vi "cBRS Readout.vi"() -> ()   [LabVIEW 2018]
uses:
  <vilib>/Utility/error.llb/DialogType.ctl
  <vilib>/DAQmx/read.llb/DAQmx Read (Analog 1D Wfm NChan NSamp).vi
  <vilib>/DAQmx/write.llb/DAQmx Write (Analog DBL 1Chan 1Samp).vi
  <vilib>/DAQmx/create/channels.llb/DAQmx Create Channel (AI-Voltage-Basic).vi
  <vilib>/DAQmx/configure/timing.llb/DAQmx Timing (Sample Clock).vi
  <vilib>/DAQmx/create/channels.llb/DAQmx Create Channel (AO-Voltage-Basic).vi
  <vilib>/DAQmx/miscellaneous.llb/DAQmx Fill In Error Info.vi
panel:
  in  "Capacitor Feedback":bool
  in  "Piezo Feedback":bool
  in  "Gain 1":dbl
  in  "Physical Channel 5":tag="Dev1/ao3" caption="Physical Channel"
  in  "Physical Channel 4":tag="Dev1/ao2" caption="Physical Channel"
  in  "I Reset 2":bool
  in  "I Reset 1":bool
  in  "To Disk Freq":dbl=500.0 caption="dt"
  in  "DC Offset 2":dbl
  in  "I term 2":dbl=5000.0
  in  "Gain 2":dbl=0.005
  in  "Setpoint 2":dbl=5.0
  in  "Physical Channel 3":tag="Dev1/ao1" caption="Physical Channel"
  in  "I term":dbl=5000.0
  in  "Output terminal configuration":i32(ring)=10083 items=["Default"=-1, "RSE"=10083, "Differential"=10106, "Pseudodifferential"=12529]
  in  "DC Offset":dbl
  in  "Gain":dbl=0.005
  in  "Setpoint":dbl=5.0
  in  "Physical Channel 2":tag="Dev1/ao0" caption="Physical Channel"
  in  "Input terminal configuration":i32(ring)=10106 items=["default"=-1, "RSE"=10083, "NRSE"=10078, "Differential"=10106, "Pseudodifferential"=12529]
  in  "Down Sample Freq":dbl=1000.0 caption="dt"
  out "Waveform Chart":dynamicdata(graph)=[{"t0"=timestamp(3662756182.4372287 s since 1904-01-01), "dt"=1.9999999999999998e-05, "Y"=array[500 elements], "attributes"=variant("NI_ChannelName"=variant(string "Dev1/ai0"), "NI_UnitDescription"=variant(string "Volts"))}, {"t0"=timestamp(3662756182.4372387 s since 1904-01-01), "dt"=1.9999999999999998e-05, "Y"=array[500 elements], "attributes"=variant("NI_ChannelName"=variant(string "Dev1/ai2"), "NI_UnitDescription"=variant(string "Volts"))}, {"t0"=timestamp(3662756182.4372287 s since 1904-01-01), "dt"=0.001, "Y"=[0.0, 0.0, 0.0, 0.0, 0.0, 0.0, 0.0, 0.0, 0.0, 0.0], "attributes"=variant("NI_ChannelName"=variant(string "Dev1/ai0 (Filtered)"), "NI_OriginalChannelName"=variant(string "Dev1/ai0"), "NI_UnitDescription"=variant(string "Volts"))}, {"t0"=timestamp(3662756182.4372287 s since 1904-01-01), "dt"=0.001, "Y"=[0.0, 0.0, 0.0, 0.0, 0.0, 0.0, 0.0, 0.0, 0.0, 0.0], "attributes"=variant("NI_ChannelName"=variant(string "Dev1/ai2 (Filtered)"), "NI_OriginalChannelName"=variant(string "Dev1/ai2"), "NI_UnitDescription"=variant(string "Volts"))}, {"t0"=timestamp(3662756182.4372287 s since 1904-01-01), "dt"=0.001, "Y"=[3.746254926547408, 3.7462550457566977, 3.7462551556527615, 3.746255255304277, 3.7462553502991796, 3.746255445294082, 3.7462555365636945, 3.7462556241080165, 3.7462557135149837, 3.7462558085098863], "attributes"=variant("NI_ChannelName"=variant(string "Dev1/ai0 (Filtered)"), "NI_OriginalChannelName"=variant(string "Dev1/ai0"), "NI_UnitDescription"=variant(string "Volts"))}]
  in  "Write":bool caption="Enable"
  in  "stop":bool
  in  "Samples to Read":i32=500
  in  "Sample Rate":dbl=50000.0 caption="Read Rate (Hz)" format="%0.2f"
  in  "Physical Channel":tag="Dev1/ai0, Dev1/ai2" caption="Input Physical Channel"
  # "Piezo Feedback 1"
  # "Piezo Feedback 2"
  # "Capacitor Feedback"
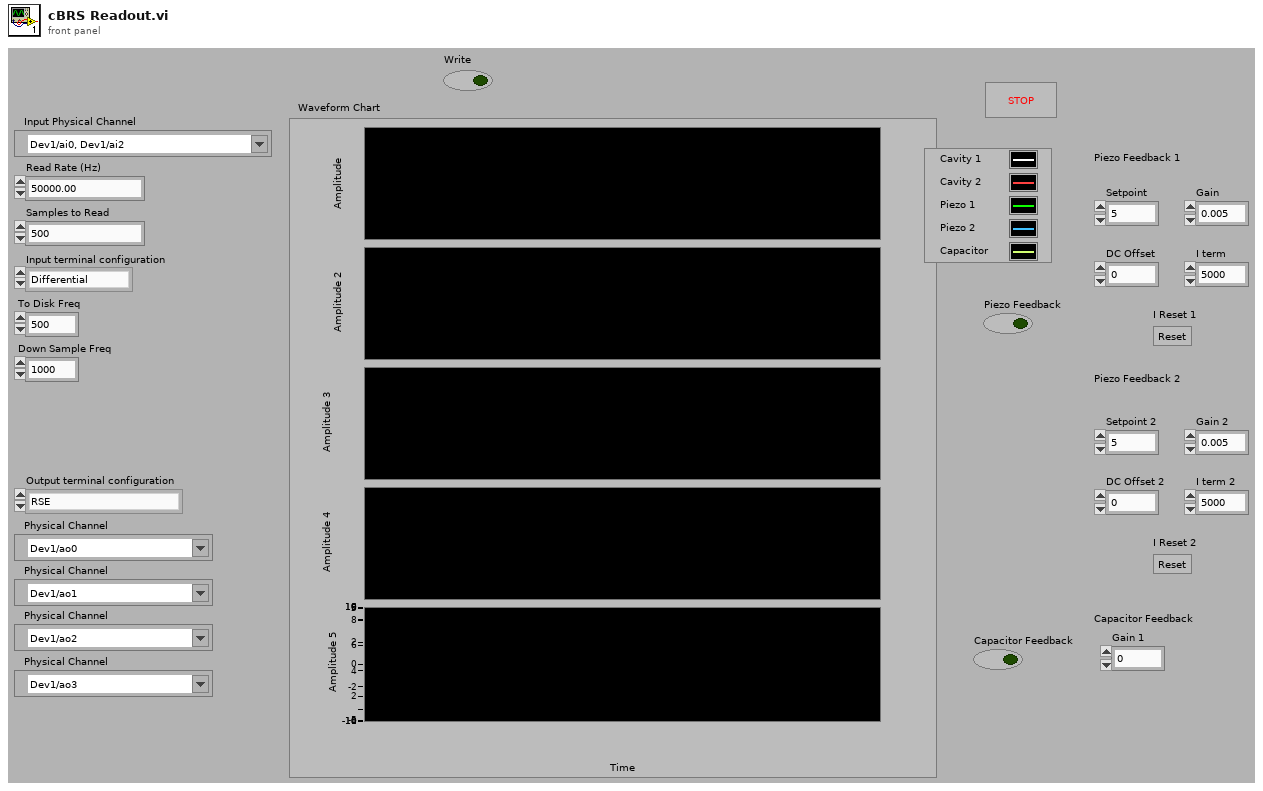
[diagram p1: front panel]
types:
  T1 = typedef "DialogType.ctl" = u16
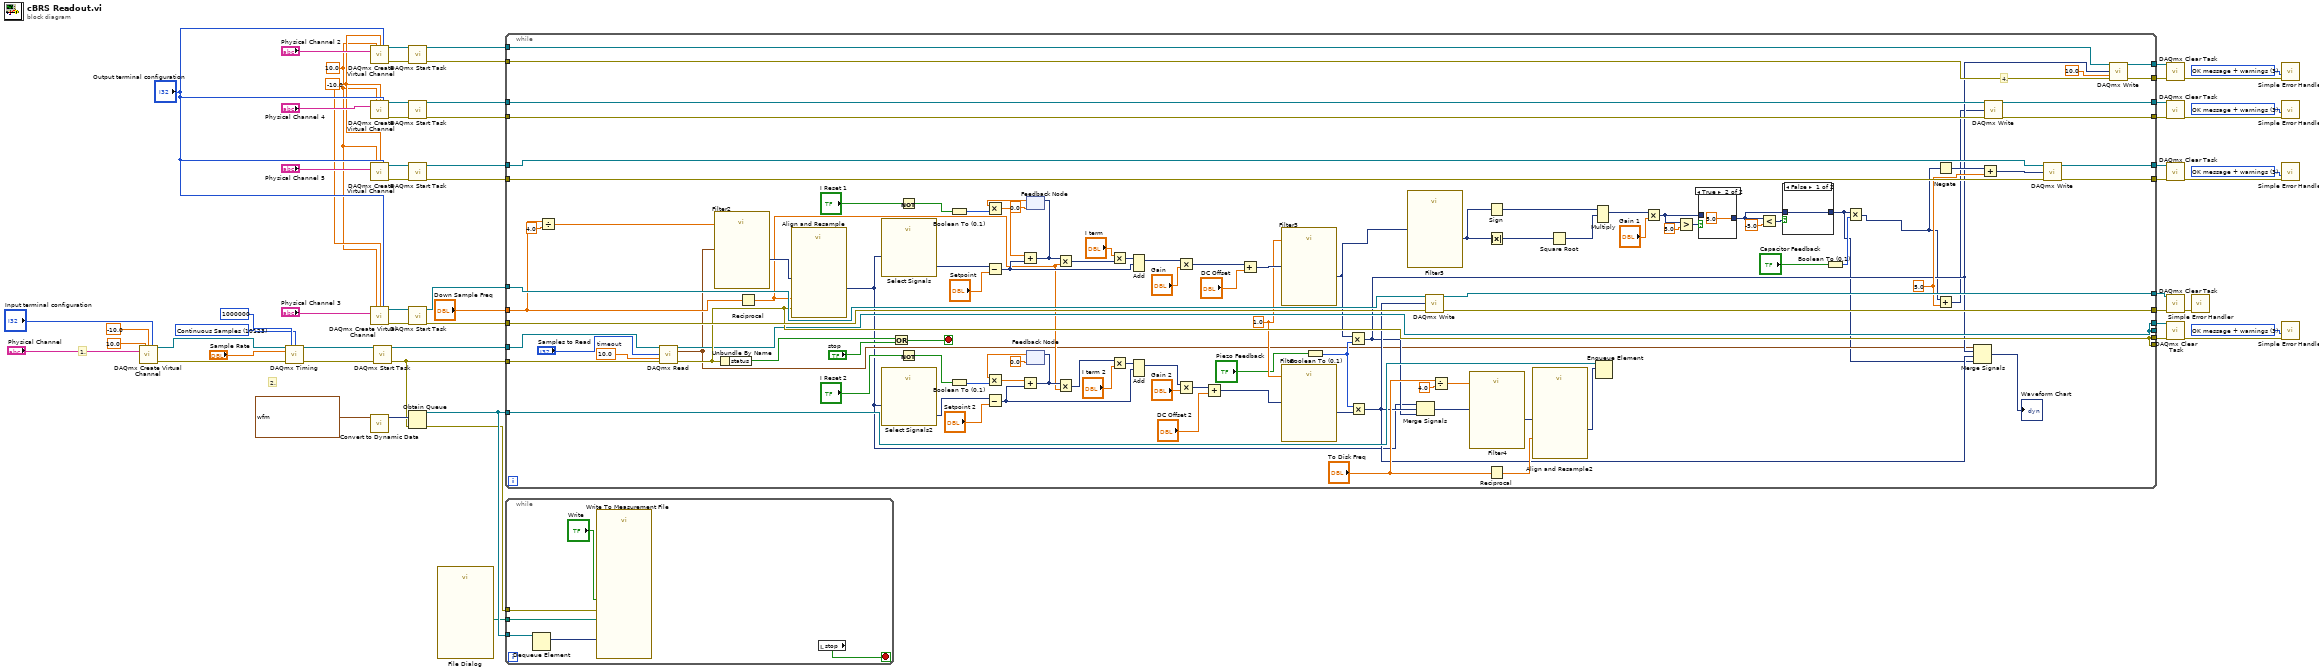
[diagram p0: block diagram]
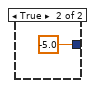
[diagram p2: hidden frame]
diagram:
  w2 = 10.0 ("maximum value")
  w3 = -10.0 ("Minimum Value 4")
  w14 = T1 3 items=["no dialog", "OK message", "continue or stop message", "OK message + warnings", "continue/stop + warnings"] ("type of dialog (OK msg:1)")
  w16 = T1 3 items=["no dialog", "OK message", "continue or stop message", "OK message + warnings", "continue/stop + warnings"] ("type of dialog (OK msg:1)")
  w44 = T1 3 items=["no dialog", "OK message", "continue or stop message", "OK message + warnings", "continue/stop + warnings"] ("type of dialog (OK msg:1)")
  w52 = T1 3 items=["no dialog", "OK message", "continue or stop message", "OK message + warnings", "continue/stop + warnings"] ("type of dialog (OK msg:1)")
  w57 = 10123 items=["Finite Samples"=10178, "Continuous Samples"=10123] ("sample mode")
  # "2."
  # "1."
  n1 = call-poly <vilib>:"DAQmx Create Virtual Channel.vi"("maximum value"=10.0, "minimum value"=-10.0 ("Minimum Value"), "input terminal configuration"="Input terminal configuration", "physical channels"="Physical Channel") -> ("task out"=w59:refnum<k21>, "error out"=w61:errorcluster)  [unwired: 10 in]
  n2 = call-poly <vilib>:"DAQmx Timing.vi"("task/channels in"=w59, "sample mode"=w57, "samples per channel"=1000000, "rate"="Sample Rate", "error in"=w61) -> ("task out"=w56:refnum<k21>, "error out"=w55:errorcluster)  [unwired: 9 in]
  n3 = call-poly <vilib>:"DAQmx Create Virtual Channel.vi"("maximum value"=w2, "minimum value"=w3, "output terminal configuration"="Output terminal configuration", "physical channels"="Physical Channel 2") -> ("task out"=w43:refnum<k21>, "error out"=w42:errorcluster)  [unwired: 10 in]
  n4 = call-poly <vilib>:"DAQmx Create Virtual Channel.vi"("maximum value"=w2, "minimum value"=w3, "output terminal configuration"="Output terminal configuration", "physical channels"="Physical Channel 4") -> ("task out"=w23:refnum<k21>, "error out"=w22:errorcluster)  [unwired: 10 in]
  n5 = call-poly <vilib>:"DAQmx Create Virtual Channel.vi"("maximum value"=w2, "minimum value"=w3, "output terminal configuration"="Output terminal configuration", "physical channels"="Physical Channel 5") -> ("task out"=w20:refnum<k21>, "error out"=w19:errorcluster)  [unwired: 10 in]
  n6 = call-poly <vilib>:"DAQmx Create Virtual Channel.vi"("maximum value"=w2, "minimum value"=w3, "output terminal configuration"="Output terminal configuration", "physical channels"="Physical Channel 3") -> ("task out"=w36:refnum<k21>, "error out"=w35:errorcluster)  [unwired: 10 in]
  n7 = call "Convert to Dynamic Data"("Waveform"=waveform(dbl) {"t0"=timestamp(0 s since 1904-01-01), "dt"=1.0, "Y"=[]}) -> ("Dynamic Data Type"=w29:dynamicdata)  [unwired: 3 in]
  n8 = call <vilib>:"DAQmx Start Task.vi"("task/channels in"=w56, "error in"=w55) -> ("task out"=w51:refnum<k21>, "error out"=w27:errorcluster)  [unwired: 12 in]
  n9 = call <vilib>:"DAQmx Start Task.vi"("task/channels in"=w43, "error in"=w42) -> ("task out"=w41:refnum<k21>, "error out"=w40:errorcluster)  [unwired: 12 in]
  n10 = call <vilib>:"DAQmx Start Task.vi"("task/channels in"=w23, "error in"=w22) -> ("task out"=w18:refnum<k21>, "error out"=w9:errorcluster)  [unwired: 12 in]
  n11 = call <vilib>:"DAQmx Start Task.vi"("task/channels in"=w20, "error in"=w19) -> ("task out"=w8:refnum<k21>, "error out"=w7:errorcluster)  [unwired: 12 in]
  n12 = call <vilib>:"DAQmx Start Task.vi"("task/channels in"=w36, "error in"=w35) -> ("task out"=w34:refnum<k21>, "error out"=w33:errorcluster)  [unwired: 12 in]
  n13 = Obtain Queue(element data type=w29, error in (no error)=w27) -> (queue out=w26:refnum<queue>, error out=w25:errorcluster)  [unwired: 3 in, 1 out]
  n14 = call "File Dialog"() -> ("selected path"=w1:path)  [unwired: 12 in, 3 out]
  n15 = while {
    tunnel: w27 -> [w166]
    tunnel: w51 -> [w165]
    tunnel: [w118] -> w50
    tunnel: [w119] -> w54
    tunnel: "Down Sample Freq" -> [w91]
    tunnel: w41 -> [w161]
    tunnel: w40 -> [w160]
    tunnel: [w159] -> w39
    tunnel: [w158] -> w38
    tunnel: w34 -> [w139]
    tunnel: w33 -> [w138]
    tunnel: [w148] -> w32
    tunnel: [w147] -> w30
    tunnel: [w119] -> _
    tunnel: [w118] -> _
    tunnel: w26 -> [w116]
    tunnel: w18 -> [w108]
    tunnel: [w107] -> w13
    tunnel: [w106] -> w12
    tunnel: [w105] -> w11
    tunnel: [w104] -> w10
    tunnel: w9 -> [w103]
    tunnel: w8 -> [w102]
    tunnel: w7 -> [w101]
    stop <- w114 stop-if-true
    w82 = 5.0 ("y")
    w109 = 1.0
    w162 = 10.0  # timeout
    # "4."
    n16 = Divide(x=w91, y=4.0) -> (x/y=w90:dbl)
    n17 = call-poly <vilib>:"DAQmx Read.vi"("task/channels in"=w165, "number of samples per channel"="Samples to Read", "timeout"=w162, "error in"=w166) -> ("task out"=w118:refnum<k21>, "data"=w71:waveform(dbl)[], "error out"=w119:errorcluster)  [unwired: 9 in]
    n18 = call "Filter2"("Lower Cut-Off"=w90, "Signal"=w71) -> ("Filtered Signal"=w154:dynamicdata)  [unwired: 8 in, 1 out]
    n19 = Unbundle By Name(w119) -> ("status"=w164:bool)
    n20 = Reciprocal(x=w91) -> (1/x=w97:dbl)
    n21 = call "Align and Resample"("dt"=w97, "error in (no error)"=w119, "Signals"=w154) -> ("Resampled Signals"=w70:dynamicdata)  [unwired: 6 in, 2 out]
    n22 = call "Select Signals"("Signals"=w70) -> ("Signal Out"=w153:dynamicdata)  [unwired: 9 in, 1 out]
    n23 = call "Select Signals2"("Signals"=w70) -> ("Signal Out"=w117:dynamicdata)  [unwired: 9 in, 1 out]
    n24 = Or(x=w164, y="stop") -> (x .or. y?=w114:bool)
    n25 = Not(x="I Reset 1") -> (.not. x?=w128:bool)
    n26 = Not(x="I Reset 2") -> (.not. x?=w122:bool)
    n27 = Boolean To (0,1)(Boolean=w128) -> (0, 1=w132:i16)
    n28 = Boolean To (0,1)(Boolean=w122) -> (0, 1=w126:i16)
    n29 = Subtract(x=w153, y="Setpoint") -> (x-y=w113:dynamicdata)
    n30 = Subtract(x=w117, y="Setpoint 2") -> (x-y=w112:dynamicdata)
    n31 = feedback #1(0.0) -> (w131:dbl)
    n32 = Multiply(x=w131, y=w132) -> (x*y=w130:dbl)
    n33 = Add(x=w130, y=w113) -> (x+y=w134:dynamicdata)
    n34 = feedback-in #1(w134) -> ()
    n35 = feedback #2(0.0) -> (w125:dbl)
    n36 = Multiply(x=w125, y=w126) -> (x*y=w124:dbl)
    n37 = Add(x=w124, y=w112) -> (x+y=w121:dynamicdata)
    n38 = feedback-in #2(w121) -> ()
    n39 = Multiply(x=w134, y=w97) -> (x*y=w135:dynamicdata)
    n40 = Multiply(x=w121, y=w97) -> (x*y=w120:dynamicdata)
    n41 = Multiply(x="I term", y=w135) -> (x*y=w151:dynamicdata)
    n42 = Multiply(x=w120, y="I term 2") -> (x*y=w144:dynamicdata)
    n43 = Add(1:w113, 2:w151) -> (0:w146:dynamicdata)  [unwired: 1 in, 1 out]
    n44 = Add(1:w112, 2:w144) -> (0:w142:dynamicdata)  [unwired: 1 in, 1 out]
    n45 = Multiply(x=w146, y="Gain") -> (x*y=w137:dynamicdata)
    n46 = Multiply(x=w142, y="Gain 2") -> (x*y=w136:dynamicdata)
    n47 = Add(x=w136, y="DC Offset 2") -> (x+y=w110:dynamicdata)
    n48 = Add(x=w137, y="DC Offset") -> (x+y=w111:dynamicdata)
    n49 = call "Filter3"("Lower Cut-Off"=w109, "Signal"=w111) -> ("Filtered Signal"=w63:dynamicdata)  [unwired: 8 in, 1 out]
    n50 = call "Filter"("Lower Cut-Off"=w109, "Signal"=w110) -> ("Filtered Signal"=w100:dynamicdata)  [unwired: 8 in, 1 out]
    n51 = Boolean To (0,1)(Boolean="Piezo Feedback") -> (0, 1=w89:i16)
    n52 = Multiply(x=w63, y=w89) -> (x*y=w79:dynamicdata)
    n53 = Multiply(x=w89, y=w100) -> (x*y=w80:dynamicdata)
    n54 = call "Filter5"("Signal"=w63) -> ("Filtered Signal"=w86:dynamicdata)  [unwired: 9 in, 1 out]
    n55 = Merge Signals(w70, w80, w79) -> (w78:dynamicdata)
    n56 = call-poly <vilib>:"DAQmx Write.vi"("task/channels in"=w139, "data"=w80, "error in"=w138) -> ("task out"=w147:refnum<k21>, "error out"=w148:errorcluster)  [unwired: 10 in, 1 out]
    n57 = Divide(x="To Disk Freq", y=4.0) -> (x/y=w93:dbl)
    n58 = call "Filter4"("Lower Cut-Off"=w93, "Signal"=w78) -> ("Filtered Signal"=w96:dynamicdata)  [unwired: 8 in, 1 out]
    n59 = Sign(1:w86) -> (0:w85:dynamicdata)
    n60 = Absolute Value(x=w86) -> (abs(x)=w87:dynamicdata)
    n61 = Reciprocal(x="To Disk Freq") -> (1/x=w98:dbl)
    n62 = call "Align and Resample2"("dt"=w98, "Signals"=w96) -> ("Resampled Signals"=w115:dynamicdata)  [unwired: 7 in, 2 out]
    n63 = Square Root(x=w87) -> (sqrt(x)=w84:dynamicdata)
    n64 = Multiply(1:w84, 2:w85) -> (0:w83:dynamicdata)  [unwired: 1 in, 1 out]
    n65 = Enqueue Element(queue=w116, element=w115) -> ()  [unwired: 2 in, 3 out]
    n66 = Multiply(x=w83, y="Gain 1") -> (x*y=w76:dynamicdata)
    n67 = Greater?(x=w76, y=5.0) -> (0:w75:dynamicdata)
    n68 = case shown="True" w75 {
      tunnel: [w169 5.0] -> w73
      tunnel: w76 -> [w169 _]
      frame False {
      }
      frame True {
      }
    }
    n69 = Less?(x=w73, y=-5.0) -> (x < y?=w74:dynamicdata)
    n70 = case shown="False" w74 {
      tunnel: w73 -> [w167 _]
      tunnel: [w167 -5.0] -> w64
      frame False {
      }
      frame True {
      }
    }
    n71 = Boolean To (0,1)(Boolean="Capacitor Feedback") -> (0, 1=w66:i16)
    n72 = Multiply(x=w64, y=w66) -> (x*y=w65:dynamicdata)
    n73 = Negate(x=w65) -> (-x=w81:dynamicdata)
    n74 = Add(x=w65, y=w82) -> (x+y=w68:dynamicdata)
    n75 = Merge Signals(w71, w79, w80, w64) -> (→"Waveform Chart":dynamicdata)
    n76 = Add(x=w81, y=w82) -> (x+y=w69:dynamicdata)
    n77 = call-poly <vilib>:"DAQmx Write.vi"("task/channels in"=w108, "data"=w68, "error in"=w103) -> ("task out"=w104:refnum<k21>, "error out"=w105:errorcluster)  [unwired: 10 in, 1 out]
    n78 = call-poly <vilib>:"DAQmx Write.vi"("task/channels in"=w102, "data"=w69, "error in"=w101) -> ("task out"=w107:refnum<k21>, "error out"=w106:errorcluster)  [unwired: 10 in, 1 out]
    n79 = call-poly <vilib>:"DAQmx Write.vi"("task/channels in"=w161, "data"=w79, "timeout"=10.0, "error in"=w160) -> ("task out"=w158:refnum<k21>, "error out"=w159:errorcluster)  [unwired: 9 in, 1 out]
  }
  n80 = while {
    tunnel: w26 -> [w176]
    tunnel: w25 -> [w173]
    tunnel: w1 -> [w171]
    stop <- w174 stop-if-true
    n81 = Dequeue Element(queue=w176) -> (element=w175:dynamicdata)  [unwired: 2 in, 3 out]
    n82 = call "Write To Measurement File"("Signals"=w175, "Enable"="Write", "error in (no error)"=w173, "Filename"=w171) -> ()  [unwired: 13 in, 3 out]
    n83 = local read "stop"() -> (w174:bool)
  }
  n84 = call <vilib>:"DAQmx Clear Task.vi"("task in"=w38, "error in"=w39) -> ("error out"=w46:errorcluster)  [unwired: 13 in]
  n85 = call <vilib>:"DAQmx Clear Task.vi"("task in"=w10, "error in"=w11) -> ("error out"=w17:errorcluster)  [unwired: 13 in]
  n86 = call <vilib>:"DAQmx Clear Task.vi"("task in"=w13, "error in"=w12) -> ("error out"=w15:errorcluster)  [unwired: 13 in]
  n87 = call <vilib>:"DAQmx Clear Task.vi"("task in"=w30, "error in"=w32) -> ("error out"=w31:errorcluster)  [unwired: 13 in]
  n88 = call <vilib>:"DAQmx Clear Task.vi"("task in"=w50, "error in"=w54) -> ("error out"=w60:errorcluster)  [unwired: 13 in]
  n89 = call <vilib>:"Simple Error Handler.vi"("error in (no error)"=w31) -> ()  [unwired: 4 in, 5 out]
  n90 = call <vilib>:"Simple Error Handler.vi"("type of dialog (OK msg:1)"=w44, "error in (no error)"=w46) -> ()  [unwired: 3 in, 5 out]
  n91 = call <vilib>:"Simple Error Handler.vi"("type of dialog (OK msg:1)"=w16, "error in (no error)"=w17) -> ()  [unwired: 3 in, 5 out]
  n92 = call <vilib>:"Simple Error Handler.vi"("type of dialog (OK msg:1)"=w14, "error in (no error)"=w15) -> ()  [unwired: 3 in, 5 out]
  n93 = call <vilib>:"Simple Error Handler.vi"("type of dialog (OK msg:1)"=w52, "error in (no error)"=w60) -> ()  [unwired: 3 in, 5 out]
